vi "Cam-color.vi"(0 "Image In":T2, 7 "error in":errorcluster) -> (20 "Image Out":T2, 21 "Classifier Session (Color Classification 1)":T1, 22 "Classes (Color Classification 1)":string[](array[string]), 27 "error out":errorcluster)   [LabVIEW 2018]
uses:
  <vilib>/vision/Image Controls.llb/IMAQ Image.ctl
  <vilib>/vision/Classification.llb/IMAQ Classifier Session.ctl
  <vilib>/vision/Classification.llb/IMAQ Classifier Read Options.ctl
  <vilib>/vision/NI_Vision_Development_Module.lvlib
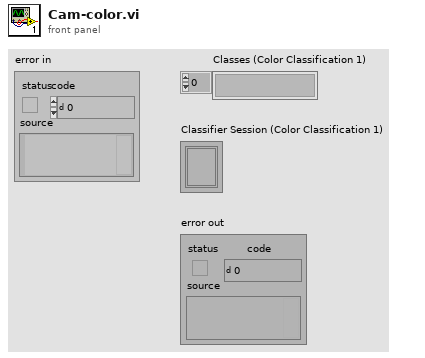
[diagram p1: front panel]
types:
  T1 = typedef "IMAQ Classifier Session.ctl" = refnum<k1>
  T2 = typedef "IMAQ Image.ctl" = refnum<image>
  T3 = cluster{"Global Rectangle":i32[], "Contours":cluster{"ID":enum32{"External", "Internal"}, "Type":u32, "Coordinates":i32[]}[]}
  T4 = typedef "IMAQ Classifier Read Options.ctl" = i32
  T5 = typedef "ROI Descriptor" = cluster{"Global Rectangle":i32[], "Contours":cluster{"ID":enum32{"External", "Internal"}, "Type":u32, "Coordinates":i32[]}[]}
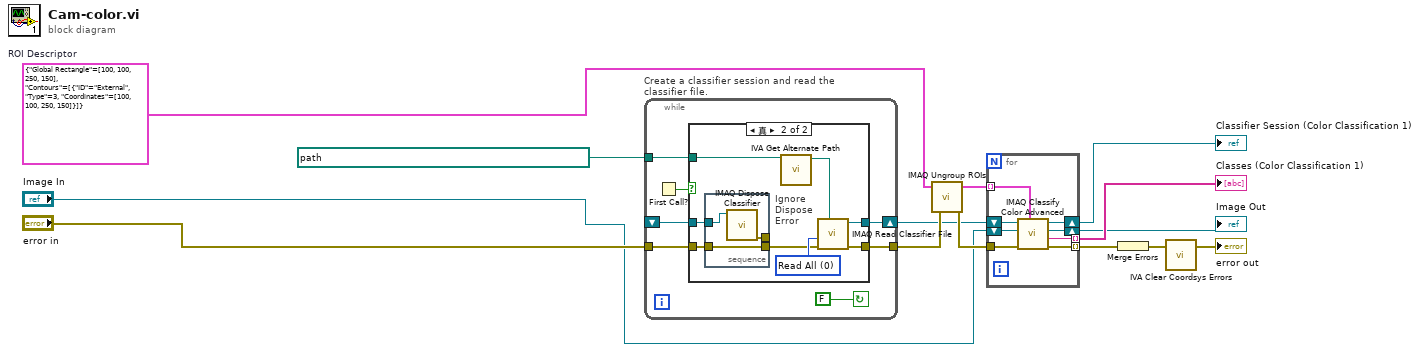
[diagram p0: block diagram]
diagram:
  w11 = T3 {"Global Rectangle"=[100, 100, 250, 150], "Contours"=[{"ID"=enum."External", "Type"=3, "Coordinates"=[100, 100, 250, 150]}]}  # ROI Descriptor
  n1 = while "Create a classifier session and read the classifier file." {
    shift-right: [w21] -> w2
    shift-left: _ -> [w20]
    tunnel: "error in" -> [w18]
    tunnel: [w17] -> w10
    tunnel: path "D:/Labviewprogram/视觉/视觉框架/Color 识别.clf" ("File Path") -> [w16]
    stop <- FALSE continue-if-true
    n2 = First Call?() -> (First Call?: T/F=w15:bool)
    n3 = case "条件结构" shown="真" w15 {
      tunnel: [w23 w30] -> w21
      tunnel: w20 -> [w23 w28]
      tunnel: w18 -> [w22 w27]
      tunnel: [w22 w29] -> w17
      tunnel: w16 -> [_ w25]
      frame False {
      }
      frame True {
        w31 = T4 0 items=["Read All", "Add Samples, Do Not Change Options", "Read Options, Do Not Add Samples"] ("Read Options")
        # "Ignore Dispose Error"
        n4 = stacked-sequence "层叠式顺序结构" {
          tunnel: w28 -> [w34]
          tunnel: w27 -> [w33]
          tunnel: [w33] -> w26
          tunnel: [w32] -> _
          frame #0 {
            n5 = call "IMAQ Dispose Classifier"("Classifier Session"=w34) -> ("error out"=w32:errorcluster)  [unwired: 1 in, 9 out]
          }
        }
        n6 = call <vilib>:"IVA Get Alternate Path.vi"("Path In"=w25) -> ("Path Out"=w24:path)  [unwired: 10 out]
        n7 = call "IMAQ Read Classifier File"("File Path"=w24, "error in (no error)"=w26, "Read Options"=w31) -> ("error out"=w29:errorcluster, "Classifier Session"=w30:T1)  [unwired: 1 in, 6 out]
      }
    }
  }
  n8 = call "IMAQ Ungroup ROIs"("error in (no error)"=w10, "ROI Descriptor"=w11) -> ("error out"=w9:errorcluster, "ROI Descriptors out"=w8:T5[])  [unwired: 2 out]
  n9 = for "For循环" {
    tunnel: [w42] -> w12 mode=indexing
    tunnel: [w41] -> w7 mode=indexing
    tunnel: w9 -> [w39]
    tunnel: w8 -> [w38] mode=indexing
    shift-right: [w36] -> w3
    shift-left: "Image In" -> [w37]
    shift-right: [w35] -> w1
    shift-left: w2 -> [w40]
    n10 = call "IMAQ Classify Color Advanced"("ROI Descriptor"=w38, "error in (no error)"=w39, "Image"=w37, "Classifier Session"=w40) -> ("error out"=w41:errorcluster, "Class"=w42:string, "Image (dup)"=w36:T2, "Classifier Session (dup)"=w35:T1)  [unwired: 4 out]
  }
  "Image Out" <- w3
  "Classes (Color Classification 1)" <- w12
  "Classifier Session (Color Classification 1)" <- w1
  n11 = Merge Errors(w7) -> (w6:errorcluster)
  n12 = call <vilib>:"IVA Clear Coordsys Errors.vi"("error in (no error)"=w6) -> ("error out"=→"error out":errorcluster)  [unwired: 10 in]
